vi "Motion_xbee_3Radars.vi"(0 "VISA resource name":refnum<visa-resource-name>="COM1", 1 "baud rate":u32=9600, 4 "data bits":u16=8 min=5 max=8 step=1, 5 "parity":u16(ring) items=["None", "Odd", "Even", "Mark", "Space"], 7 "stop bits":u16=10, 9 "XON Character":u8=17 format="%.0x", 14 "XOFF Character":u8=19 format="%.0x", 15 "timeout (ms)":u32=10000, 21 "End read on termination character?":bool, 24 "termination char\n(0xA = '\\n' = LF)":u8=10 format="%.0x", 25 "buffer size":u32=4096) -> ()   [LabVIEW 2015]
doc: "The Advanced Serial Read and Write example performs a Serial Port Read, a Serial Port Write, or a combination of these actions while setting some advanced serial features like buffer size, termination characters, and XON/XOFF flow control. The user selects the actions (read or write) on the front panel. If both are selected, the VI will write the data first, read the data and then close the VISA session that is opened to the port. \n\nThe parameters set for the serial port must match the parameters of the connected instrument or device. In this example, the bytes to read parameter specifies the number of bytes that the serial port reads. If there were more bytes at the port than the number specified in bytes to read, those bytes would not be read. Also, if you specify to read more bytes than the number of bytes actually read, you might receive a timeout error message.\n\nINSTRUCTIONS:\n1) Select the serial resource and configuration parameters (baud rate, data bits, parity, stop bits, flow control).\n2) Termination character can be enabled and set. Also, set the required input buffer size prior to running the example.\n3) Select the operations to be performed. \n4) Connect the serial port to your device. If no device is available, perform a loopback test by doing one of the following. Short pins 2 and 3 on a RS-232 cable or short pin 4 to pin 8 and pin 5 to pin 9 on a RS-485/422 cable. \n5) Run the VI to see the data read. (The \"read string\" will match the \"string to write\" if a loopback test was performed.)\n\nThis example exposes several advanced features that you may need for your application. Not all applications need all the features shown in this example. The input buffer size is likely an important setting that you want to control in your application. This example expands upon the flow control option for XON and XOFF, allowing the user to choose those control characters. The timeout parameter has been brought to the front panel so a user can specify the time period the VISA Read will wait for the number of bytes to read before timing out. Also, the user has several controls for the termination character, which is discussed later.\n\nNote that you can press the write and read buttons and change the bytes to read parameters on the fly, while the example is running. However, you must stop the example to change the other configuration parameters after the example has started running, and then run again.\n\nSet the I/O buffer size slightly higher the amount of data you expect to receive. This is very important for applications that don't use flow control, as you may lose characters if the receive buffer overflows.\n\nSetting the timeout period ensures that the operation returns with a timeout error if the operation cannot be performed in the specified time period. \n\nSome devices require a termination character in order to identify the end of command strings. Some devices send a termination character to signify the end of data to be read. \n\nThis example shows how you can end the Read operation once a termination character is detected in the buffer and/or append a termination character at the end of the Write data. To enable the Read to end on a termination character, use the VISA Configure Serial Port or use the VISA Properties Serial End Mode for Reads, Termination Character Enable, and Termination Character. To end the Write with a termination character, use the VISA Properties Serial End Mode for Writes, the Send End Enable, and Termination Character. In this example, the same termination character is used for both the Read and the Write. You can specify two different characters for your application, if desired.\n\nYour application may require specific characters for the XON/XOFF Flow Control. You can specify these characters with the VISA Properties Flow Control XOFF Character and Flow Control XON Character. Note that if the standard XON and XOFF characters are used, then decimal 17 and 19 are unavailable for data values. Remember that using flow control and setting an adequate buffer size allow you to prevent buffer overflows."
uses:
  <vilib>/Instr/_visa.llb/VISA Configure Serial Port (Instr).vi
panel:
  out "I/Q":waveform(dbl)(graph)
  out "Spectrum":waveform(dbl)(graph)
  out "I/Q":waveform(dbl)(graph)
  out "Spectrum":waveform(dbl)(graph)
  out "Spectrum":waveform(dbl)(graph)
  out "I/Q channels":waveform(dbl)(graph)
  in  "Data saving path":path=path "C:/Users/zpeng/OneDrive - Texas Tech University/Desktop/BeamSteering/data"
  in  "Save raw data":bool
  in  "FFT":i32=800
  in  "flow control":u16(ring) items=["None"=0, "XON/XOFF"=1, "RTS/CTS"=2, "DTR/DSR"=4]
  # "Radar 2"
  # "Radar 3"
  # "Radar 1"
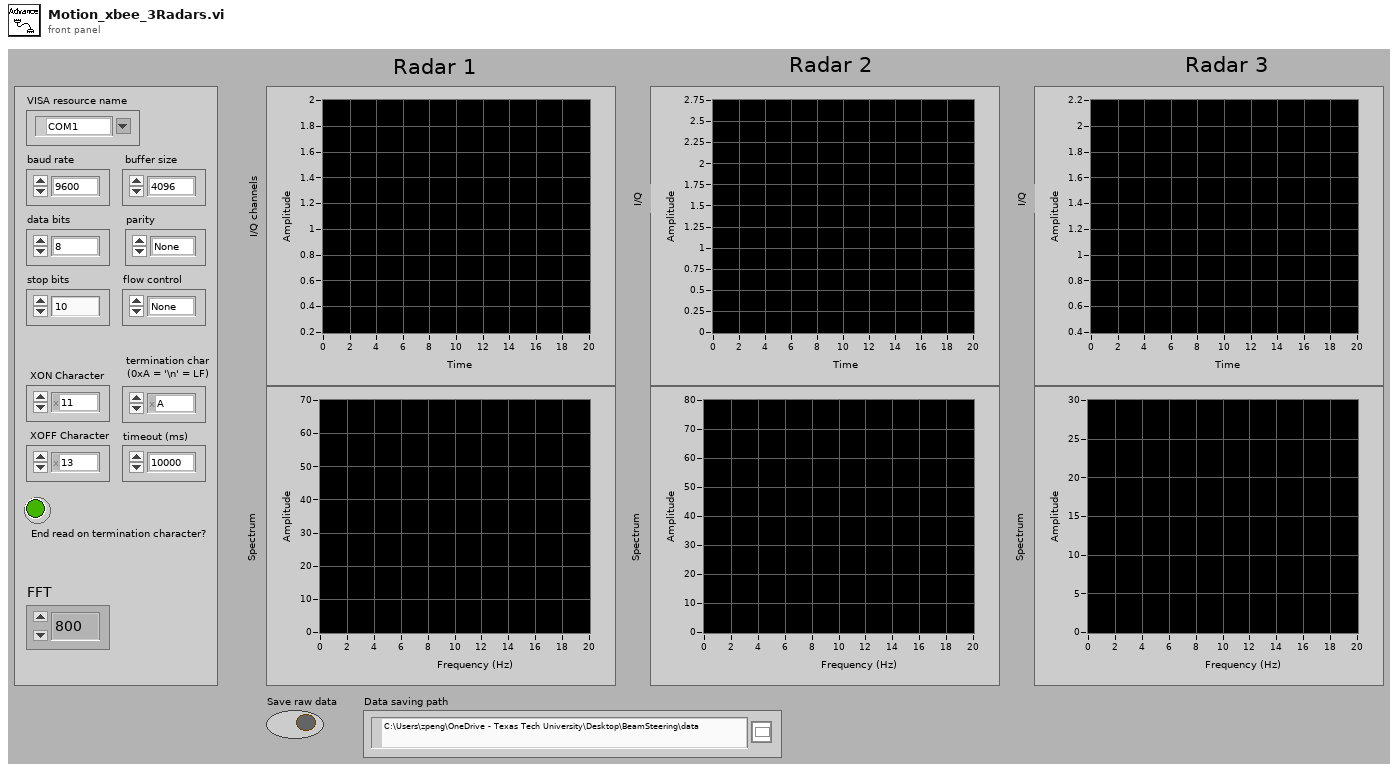
[diagram p1: front panel]
types:
  T1 = cluster{"VISA resource name out":refnum<visa-resource-name>, "error IO":errorcluster, "y":u8, i32, "Data saving path":path, "Save raw data":bool}
  T2 = cluster{"VISA resource out ":refnum<visa-resource-name>, "error out":errorcluster, "y":u8, i32, "Data saving path":path, "Save raw data":bool}
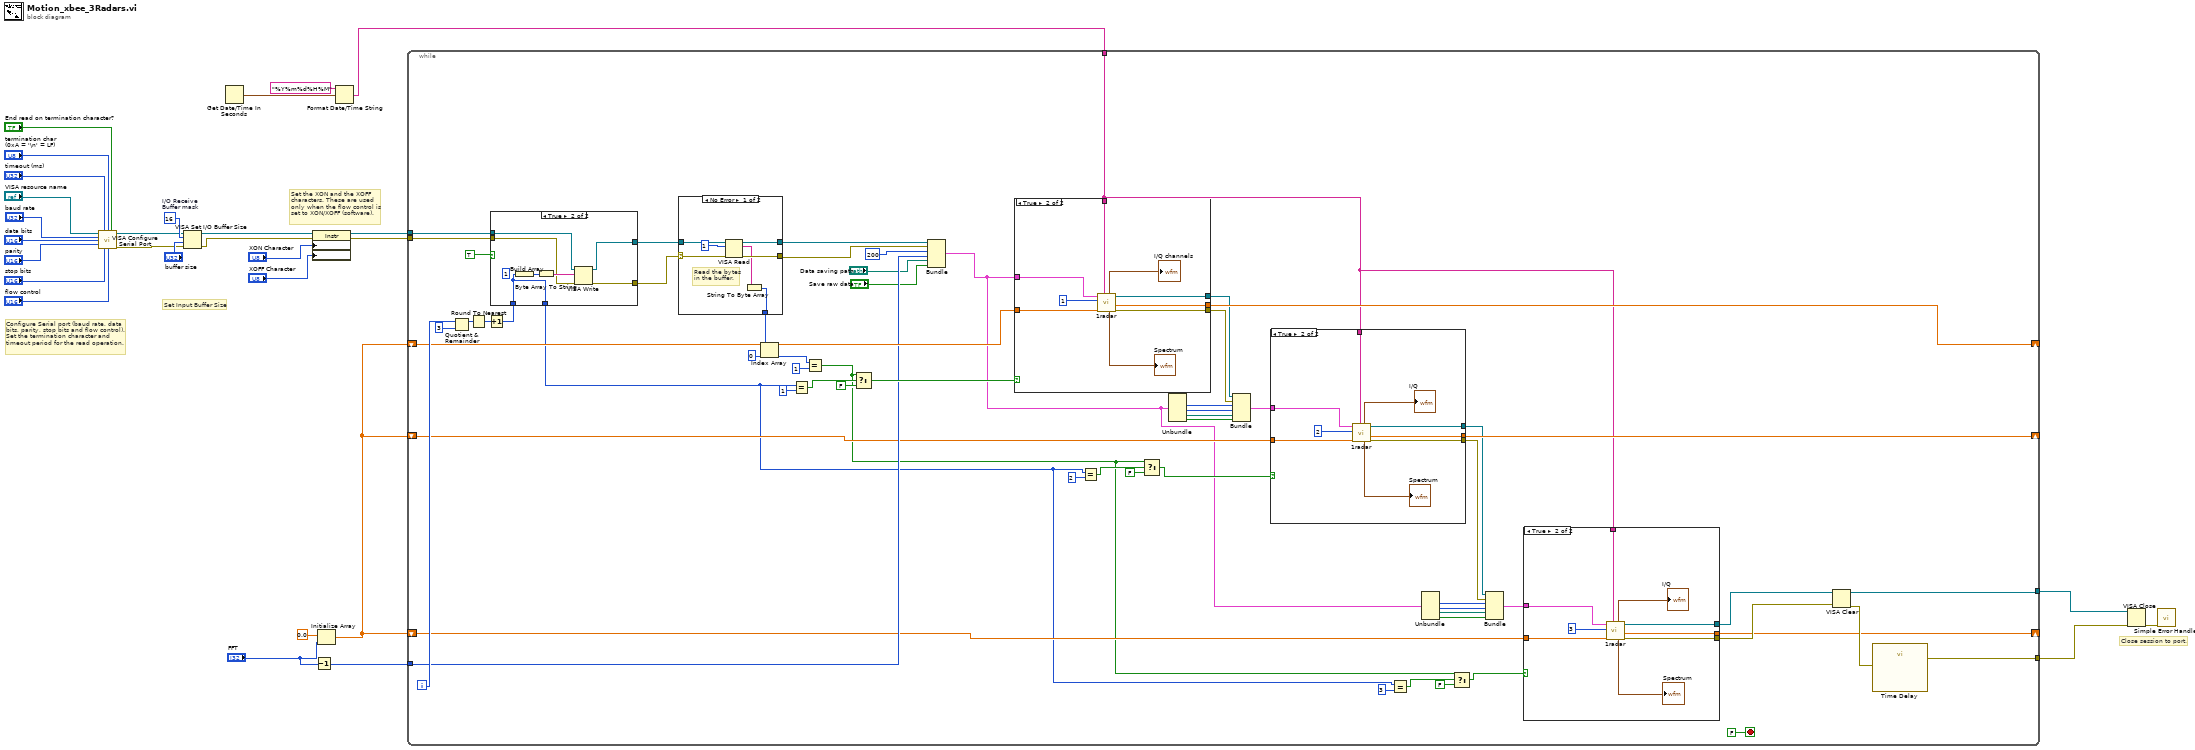
[diagram p0: block diagram]
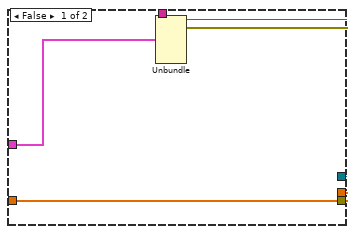
[diagram p2: hidden frame]
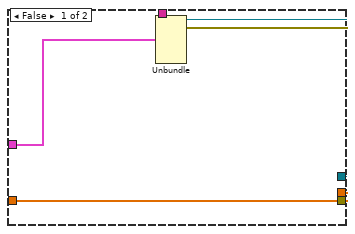
[diagram p3: hidden frame]
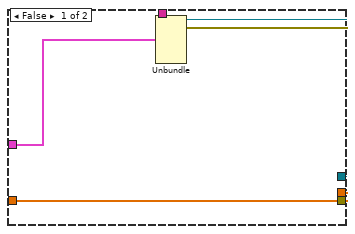
[diagram p5: hidden frame]
diagram:
  w22 = u16 16  # I/O Receive Buffer mask
  # "Set the XON and the XOFF\ncharacters. These are used\nonly when the flow control is\nset to XON/XOFF (software)."
  # "Configure Serial port (baud rate, data\nbits, parity, stop bits and flow control).\nSet the termination character and\ntimeout period for the read operation."
  # "Set Input Buffer Size"
  # "Close session to port."
  n1 = call-poly "VISA Configure Serial Port"("VISA resource name"="VISA resource name", "timeout (10sec)"="timeout (ms)", "termination char\n(0xA = '\\n' = LF)"="termination char\n(0xA = '\\n' = LF)", "Enable Termination\nChar (T)"="End read on termination character?", "baud rate (9600)"="baud rate", "data bits (8)"="data bits", "parity (0:none)"="parity", "stop bits (10: 1 bit)"="stop bits", "flow control (0:none)"="flow control") -> ("VISA resource name out"=w8:refnum<visa-resource-name>, "error out"=w7:errorcluster)  [unwired: 1 in, 4 out]
  n2 = VISA Set I/O Buffer Size(VISA resource name=w8, mask (16)=w22, size (4096)="buffer size", error in (no error)=w7) -> (VISA resource name out=w18:refnum<visa-resource-name>, error out=w17:errorcluster)
  n3 = Get Date/Time In Seconds() -> (seconds since 1Jan1904=w3:timestamp)
  n4 = property class="Instr"(reference=w18, error in=w17, "Serial Settings:Flow Control XON Character"="XON Character", "Serial Settings:Flow Control XOFF Character"="XOFF Character") -> (reference out=w6:refnum<visa-resource-name>, error out=w5:errorcluster)
  n5 = Decrement(x="FFT") -> (x-1=w11:i32)
  n6 = Initialize Array(0.0 ("element"), "FFT") -> (w1:dbl[])
  n7 = Format Date/Time String(time format string (%c)="%Y%m%d%H%M", seconds (now)=w3) -> (date/time string=w2:string)  [unwired: 1 in]
  n8 = while {
    tunnel: w11 -> [w64]
    tunnel: w6 -> [w88]
    tunnel: [w84] -> w13
    tunnel: w5 -> [w89]
    tunnel: [w86] -> w12
    shift-right: [w90] -> _
    shift-left: w1 -> [w68]
    tunnel: w2 -> [w42]
    shift-right: [w53] -> _
    shift-left: w1 -> [w56]
    shift-right: [w36] -> _
    shift-left: w1 -> [w37]
    i -> [w77]
    stop <- FALSE stop-if-true
    n9 = Quotient & Remainder(x=w77, y=3) -> (x-y*floor(x/y)=w78:i32)  [unwired: 1 out]
    n10 = Round To Nearest(number=w78) -> (nearest integer value=w75:i32)
    n11 = Increment(x=w75) -> (x+1=w72:i32)
    n12 = case shown="True" TRUE {
      tunnel: w89 -> [w142 w148]
      tunnel: w88 -> [w141 w147]
      tunnel: [w141 w146] -> w82
      tunnel: [w142 w145] -> w83
      tunnel: w72 -> [_ w143]
      tunnel: [_ w143] -> w30
      frame False {
      }
      frame True {
        (unwired) u8 1 ("element")
        n13 = Build Array(w143) -> (w144:i32[])
        n14 = Byte Array To String(unsigned byte array=w144) -> (string=w149:string)
        n15 = VISA Write(VISA resource name=w147, write buffer=w149, error in (no error)=w148) -> (VISA resource name out=w146:refnum<visa-resource-name>, error out=w145:errorcluster)  [unwired: 1 out]
      }
    }
    n16 = case "Read bytes from port." shown="No Error" w83 {
      selector: w83 -> [w121 w126]
      tunnel: [w123 w126] -> w66
      tunnel: [w124 w127] -> w67
      tunnel: w82 -> [w122 w127]
      tunnel: [w119 u8[] [] ("unsigned byte array")] -> w81
      frame No Error {
        # "Read the bytes\nin the buffer."
        n17 = VISA Read(VISA resource name=w122, byte count=u32 1, error in (no error)=w121) -> (VISA resource name out=w124:refnum<visa-resource-name>, read buffer=w120:string, error out=w123:errorcluster)  [unwired: 1 out]
        n18 = String To Byte Array(string=w120) -> (unsigned byte array=w119:u8[])
      }
      frame Error {
        # "Error occurred \nreading Bytes at \nSerial Port"
      }
    }
    n19 = Index Array(array=w81, index=0) -> (element=w79:u8)
    n20 = Equal?(x=w30, y=1) -> (x = y?=w70:bool)
    n21 = Equal?(x=w79, y=u8 1) -> (x = y?=w31:bool)
    n22 = Select(t=w31, s=w70, f=FALSE) -> (s? t:f=w74:bool)
    n23 = Bundle("VISA resource name out"=w67, "error IO"=w66, "y"=u8 200, w64, "Data saving path"="Data saving path", "Save raw data"="Save raw data") -> (w44:T1)  [unwired: 1 in]
    n24 = case shown="True" w74 {
      tunnel: [w131 w135] -> w90
      tunnel: [w129 w137] -> w55
      tunnel: [w128 w136] -> w54
      tunnel: w42 -> [_ w134]
      tunnel: w68 -> [w131 w138]
      tunnel: w44 -> [w130 w140]
      frame False {
        n25 = Unbundle(w130) -> ("VISA resource name out"=w129:refnum<visa-resource-name>, "error IO"=w128:errorcluster)  [unwired: 4 out]
      }
      frame True {
        n26 = call "1radar.vi"("date/time string"=w134, "Q"=w138, "radar number"=u8 1 ("y"), "input cluster"=w140) -> ("error out"=w136:errorcluster, "Q out"=w135:dbl[], "VISA resource out"=w137:refnum<visa-resource-name>, "Spectrum"=→"Spectrum":waveform(dbl), "I/Q channels"=→"I/Q channels":waveform(dbl))  [unwired: 3 in]
      }
    }
    n27 = Equal?(x=w30, y=2) -> (x = y?=w52:bool)
    n28 = Select(t=w31, s=w52, f=FALSE) -> (s? t:f=w49:bool)
    n29 = Unbundle(w44) -> ("y"=w61:u8, w60:i32, "Data saving path"=w59:path, "Save raw data"=w58:bool)  [unwired: 2 out]
    n30 = Bundle("VISA resource out"=w55, "error out"=w54, "y"=w61, w60, "Data saving path"=w59, "Save raw data"=w58) -> (w57:T2)  [unwired: 1 in]
    n31 = case shown="True" w49 {
      tunnel: [w108 w112] -> w53
      tunnel: [w106 w114] -> w41
      tunnel: [w105 w113] -> w39
      tunnel: w42 -> [_ w111]
      tunnel: w56 -> [w108 w115]
      tunnel: w57 -> [w107 w117]
      frame False {
        n32 = Unbundle(w107) -> ("VISA resource out"=w106:refnum<visa-resource-name>, "error out"=w105:errorcluster)  [unwired: 4 out]
      }
      frame True {
        n33 = call "1radar.vi"("date/time string"=w111, "Q"=w115, "radar number"=u8 2 ("y"), "input cluster"=w117) -> ("error out"=w113:errorcluster, "Q out"=w112:dbl[], "VISA resource out"=w114:refnum<visa-resource-name>, "Spectrum"=→"Spectrum":waveform(dbl), "I/Q channels"=→"I/Q":waveform(dbl))  [unwired: 3 in]
      }
    }
    n34 = Equal?(x=w30, y=3) -> (x = y?=w35:bool)
    n35 = Unbundle(w44) -> ("y"=w48:u8, w47:i32, "Data saving path"=w46:path, "Save raw data"=w45:bool)  [unwired: 2 out]
    n36 = Select(t=w31, s=w35, f=FALSE) -> (s? t:f=w32:bool)
    n37 = Bundle("VISA resource out"=w41, "error out"=w39, "y"=w48, w47, "Data saving path"=w46, "Save raw data"=w45) -> (w43:T2)  [unwired: 1 in]
    n38 = case shown="True" w32 {
      tunnel: [w95 w99] -> w36
      tunnel: [w93 w101] -> w40
      tunnel: [w92 w100] -> w38
      tunnel: w42 -> [_ w98]
      tunnel: w37 -> [w95 w102]
      tunnel: w43 -> [w94 w104]
      frame False {
        n39 = Unbundle(w94) -> ("VISA resource out"=w93:refnum<visa-resource-name>, "error out"=w92:errorcluster)  [unwired: 4 out]
      }
      frame True {
        n40 = call "1radar.vi"("date/time string"=w98, "Q"=w102, "radar number"=u8 3 ("y"), "input cluster"=w104) -> ("error out"=w100:errorcluster, "Q out"=w99:dbl[], "VISA resource out"=w101:refnum<visa-resource-name>, "Spectrum"=→"Spectrum":waveform(dbl), "I/Q channels"=→"I/Q":waveform(dbl))  [unwired: 3 in]
      }
    }
    n41 = VISA Clear(VISA resource name=w40, error in (no error)=w38) -> (VISA resource name out=w84:refnum<visa-resource-name>, error out=w85:errorcluster)
    n42 = call "Time Delay"("error in (no error)"=w85) -> ("error out"=w86:errorcluster)  [unwired: 10 in]
  }
  n43 = VISA Close(VISA resource name=w13, error in (no error)=w12) -> (error out=w27:errorcluster)
  n44 = call <vilib>:"Simple Error Handler.vi"("error in (no error)"=w27) -> ()  [unwired: 1 in, 8 out]
